vi "Begin.vi"(8 "error in":errorcluster) -> (0 "error out":errorcluster)   [LabVIEW 2020]
doc: "Called before other user functions, this VI is expected to open initial I/O refnums, load in file data, and do all program initialization. Notice that the <B>error out</B> terminal is simply used for data flow. Wiring it to other structures or subVIs ensures that this VI runs first."
uses:
  <vilib>/Rock Robotics/WPI/DriverStation/WPI_DriverStationRobotMode2.ctl
  <vilib>/Rock Robotics/WPI/Joystick/WPI_JoystickDeviceEnum.ctl
  <vilib>/Rock Robotics/WPI/Solenoid/WPI_SolenoidChannel.ctl
  <vilib>/Rock Robotics/WPI/ThirdParty/Phoenix-LabVIEW/Motor Controller/Controls/CTRE_Phoenix_MotorControl_NeutralMode.ctl
  <vilib>/Rock Robotics/SystemInterfaces/DIO/FPGA_DIOChannel.ctl
  Status Frame Stuff/Talon Status Config Array.ctl
  Status Frame Stuff/Talon Status Frame Setting.ctl
  <vilib>/Rock Robotics/WPI/ThirdParty/Phoenix-LabVIEW/Motor Controller/Controls/CTRE_Phoenix_MotorControl_StatusFrameEnhanced.ctl
  Status Frame Stuff/STATUS_Period.ctl
  Status Frame Stuff/Pigeon Status Config Array.ctl
  <vilib>/Rock Robotics/WPI/ThirdParty/Phoenix-LabVIEW/Pigeon IMU/CTRE_PigeonIMU_StatusFrameRate.ctl
  <vilib>/Rock Robotics/WPI/ThirdParty/REV Robotics/REVLib/Typedef/Spark MAX Idle Mode.ctl
  Robot Global Data.vi
  <vilib>/Rock Robotics/WPI/Utilities/WPI_GetSetVariantRefNum.vi
  <vilib>/Rock Robotics/WPI/Solenoid/WPI_SolenoidOpenDouble.vi
  <vilib>/Rock Robotics/WPI/ThirdParty/Phoenix-LabVIEW/Pigeon IMU/CTRE_PigeonIMU_Open_CAN.vi
panel:
  in  "Flywheel PIDF Constants":T1={"Set Constants"=TRUE, "P"=0.1, "I"=0.001, "D"=0.0, "F"=0.0461, "I Zone"=1000.0, "Cruise Velocity"=0, "Acceleration"=0, "Percent Deadband"=0.0}
  in  "Climber PIDF":T1={"Set Constants"=TRUE, "P"=0.45, "I"=0.0, "D"=0.0, "F"=0.0, "I Zone"=0.0, "Cruise Velocity"=20000, "Acceleration"=40000, "Percent Deadband"=0.7}
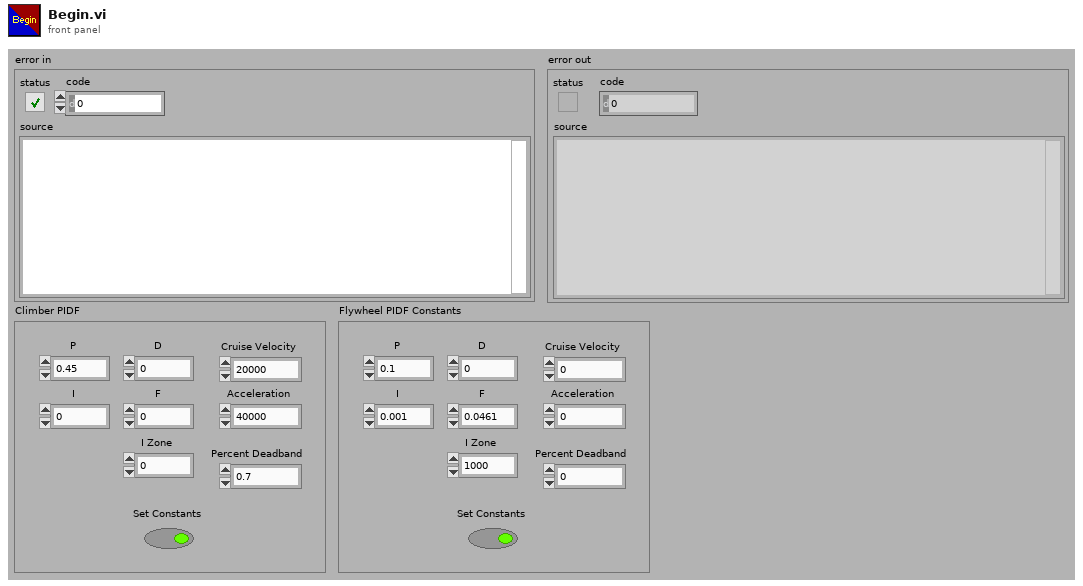
[diagram p1: front panel]
types:
  T1 = cluster{"Set Constants":bool, "P":dbl, "I":dbl, "D":dbl, "F":dbl, "I Zone":dbl, "Cruise Velocity":i32, "Acceleration":i32, "Percent Deadband":dbl}
  T2 = typedef "Pigeon Status Config Array.ctl" = cluster{"Status Frame Enum":T3, "STATUS_Period":T4}[]
  T3 = typedef "CTRE_PigeonIMU_StatusFrameRate.ctl" = u32
  T4 = typedef "STATUS_Period.ctl" = i32
  T5 = typedef "CTRE_Phoenix_MotorControl_NeutralMode.ctl" = enum8{"EEPROMSetting", "Override to Coast", "Override to Brake"}
  T6 = typedef "Talon Status Config Array.ctl" = T7[]
  T7 = typedef "Talon Status Frame Setting.ctl" = cluster{"Status Frame Enum":T8, "STATUS_Period":T4}
  T8 = typedef "CTRE_Phoenix_MotorControl_StatusFrameEnhanced.ctl" = u16
  T9 = typedef "FPGA_DIOChannel.ctl" = enum8{"DIO 0", "DIO 1", "DIO 2", "DIO 3", "DIO 4", "DIO 5", "DIO 6", "DIO 7", "DIO 8", "DIO 9", "DIO MXP 0", "DIO MXP 1", "DIO MXP 2", "DIO MXP 3", "DIO MXP 4", "DIO MXP 5", "DIO MXP 6", "DIO MXP 7", "DIO MXP 8", "DIO MXP 9", "DIO MXP 10", "DIO MXP 11", "DIO MXP 12", "DIO MXP 13", "DIO MXP 14", "DIO MXP 15", "SPI Port CS1", "SPI Port CS2", "SPI Port CS3", "SPI Port MISO", "SPI Port MOSI", "Invalid"}
  T10 = typedef "WPI_SolenoidChannel.ctl" = enum8{"Solenoid 0", "Solenoid 1", "Solenoid 2", "Solenoid 3", "Solenoid 4", "Solenoid 5", "Solenoid 6", "Solenoid 7", "Solenoid 8", "Solenoid 9", "Solenoid 10", "Solenoid 11", "Solenoid 12", "Solenoid 13", "Solenoid 14", "Solenoid 15", "Invalid"}
  T11 = typedef "WPI_JoystickDeviceEnum.ctl" = enum16{"USB 0", "USB 1", "USB 2", "USB 3", "USB 4", "USB 5"}
  T12 = typedef "WPI_DriverStationRobotMode2.ctl" = enum16{"Autonomous Disabled", "Autonomous Enabled", "Teleop Disabled", "Teleop Enabled", "Disconnected", "Finish", "Test Disabled", "Test Enabled", "Emergency Stopped"}
  T13 = typedef "WPI_JoystickDevRef.ctl" = cluster{"Device":T11}
  T14 = typedef "WPI_CompressorDevRef.ctl" = cluster{"DevStatus":errorcluster, "Pneumatics Control Module":u8}
  T15 = typedef "WPI_SolenoidDevRef.ctl" = cluster{"DevStatus":errorcluster, "Pneumatics Control Module":u8, "Forward Solenoid Channel":T10, "Reverse Solenoid Channel":T10}
  T16 = typedef "WPI_DigitalInputDevRef.ctl" = cluster{"DevStatus":errorcluster, "DIO Channel":T9}
  T17 = typedef "CTRE_PigeonIMU_DeviceRef.ctl" = cluster{"DeviceStatus":errorcluster, "Device Number":u8, "Type":T18, "Device ID":u32, "Handle":u64, "UsageFrame":u32, "Library Path":path}
  T18 = typedef "CTRE_PigeonIMU_ConnectionType.ctl" = u32
  T19 = typedef "WPI_MotorControlDeviceRef.ctl" = cluster{"DeviceStatus":errorcluster, "Type":T20, "PWM":cluster{"PWM Channel":T21, "DeadBand":T22}, "CAN":cluster{"Device Number":u8, "SetOutput VI Ref":variant, "GetOutput VI Ref":variant, "Enable VI Ref":variant, "Disable VI Ref":variant, "Data":variant}, "Invert":bool, "DIO PWM":cluster{"PWM \"Enable\" Channel":T21, "DIOChannel":T9, "PWM Rate":dbl}}
  T20 = typedef "WPI_MotorControlType.ctl" = enum16{"PWM", "CAN", "DIO PWM"}
  T21 = typedef "FPGA_DIOPWMChannel.ctl" = enum8{"PWM 0", "PWM 1", "PWM 2", "PWM 3", "PWM 4", "PWM 5", "PWM 6", "PWM 7", "PWM 8", "PWM 9", "PWM MXP 0", "PWM MXP 1", "PWM MXP 2", "PWM MXP 3", "PWM MXP 4", "PWM MXP 5", "PWM MXP 6", "PWM MXP 7", "PWM MXP 8", "PWM MXP 9", "Invalid"}
  T22 = typedef "WPI_PWMDeadband.ctl" = cluster{"Name":string, "maxPositivePwm":i32, "minPositivePwm":i32, "centerPwm":i32, "maxNegativePwm":i32, "minNegativePwm":i32, "angularRange":u16}
  T23 = typedef "Spark MAX Idle Mode.ctl" = enum16{"Coast", "Brake"}
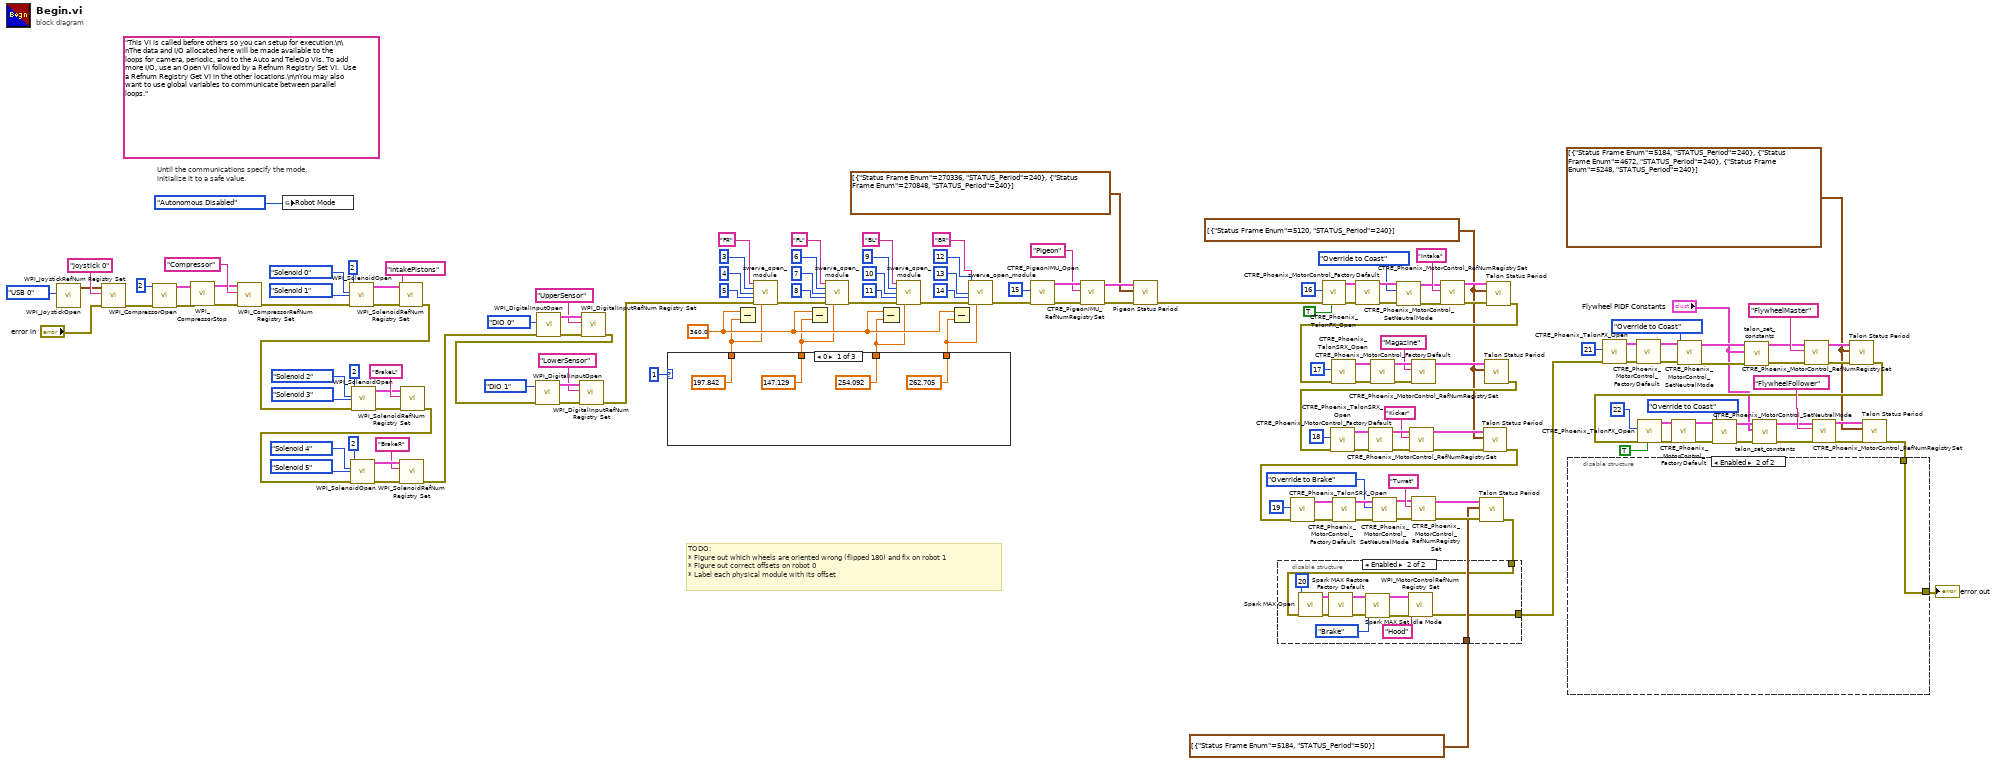
[diagram p0: block diagram]
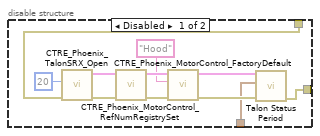
[diagram p2: hidden frame]
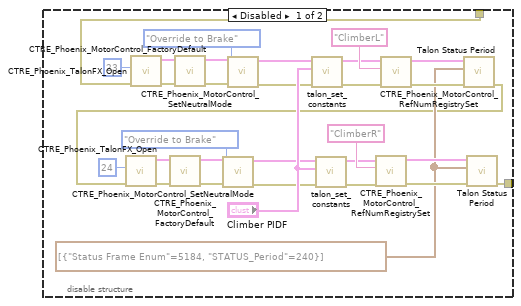
[diagram p3: hidden frame]
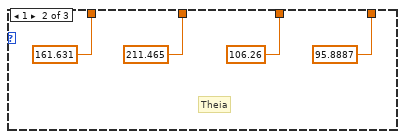
[diagram p4: hidden frame]
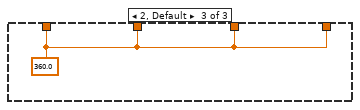
[diagram p5: hidden frame]
diagram:
  w30 = T6 [{"Status Frame Enum"=5184, "STATUS_Period"=240}, {"Status Frame Enum"=4672, "STATUS_Period"=240}, {"Status Frame Enum"=5248, "STATUS_Period"=240}] ("Drive Status Config")
  w31 = T6 [{"Status Frame Enum"=5184, "STATUS_Period"=50}] ("Drive Status Config")
  w32 = T6 [{"Status Frame Enum"=5120, "STATUS_Period"=240}] ("Drive Status Config")
  w127 = 360.0 ("Encoder Offset (Deg)")
  (unwired) "This VI is called before others so you can setup for execution.\n\nThe data and I/O allocated here will be made available to the loops for camera, periodic, and to the Auto and TeleOp VIs. To add more I/O, use an Open VI followed by a Refnum Registry Set VI.  Use a Refnum Registry Get VI in the other locations.\n\nYou may also want to use global variables to communicate between parallel loops."
  # "TODO:\n* Figure out which wheels are oriented wrong (flipped 180) and fix on robot 1\n* Figure out correct offsets on robot 0\n* Label each physical module with its offset"
  # "Until the communications specify the mode,\ninitialize it to a safe value."
  n1 = call <vilib>:"WPI_JoystickOpen.vi"("JoystickDevice"=WPI_JoystickDeviceEnum."USB 0") -> ("JoystickDevRef"=w153:T13)  [unwired: 10 in]
  n2 = call <vilib>:"WPI_JoystickRefNum Registry Set.vi"("error in (no error)"="error in", "refnum name"="Joystick 0", "JoystickDevRef"=w153) -> ("error out"=w71:errorcluster)  [unwired: 7 in, 1 out]
  n3 = call <vilib>:"WPI_CompressorOpen.vi"("Pneumatics device (def)"=u8 2, "error in (no error)"=w71) -> ("CompressorDevRef"=w24:T14, "error out"=w25:errorcluster)  [unwired: 12 in]
  n4 = call <vilib>:"WPI_CompressorStop.vi"("error in (no error)"=w25, "CompressorDevRef"=w24) -> ("error out"=w22:errorcluster, "CompressorDevRef"=w23:T14)  [unwired: 8 in]
  n5 = call <vilib>:"WPI_CompressorRefNum Registry Set.vi"("error in (no error)"=w22, "refnum name"="Compressor", "CompressorDevRef"=w23) -> ("error out"=w69:errorcluster)  [unwired: 7 in, 1 out]
  n6 = global write "Robot Global Data.vi" "Robot Mode"(WPI_DriverStationRobotMode2."Autonomous Disabled" ("Robot Mode")) -> ()
  n7 = call-poly <vilib>:"WPI_SolenoidOpen.vi"("error in (no error)"=w69, "Reverse Solenoid Channel"=WPI_SolenoidChannel."Solenoid 1", "Forward Solenoid Channel"=WPI_SolenoidChannel."Solenoid 0", "Pneumatics Device (def)"=u8 2) -> ("error out"=w126:errorcluster, "SolenoidDevRef"=w125:T15)  [unwired: 6 in]
  n8 = call <vilib>:"WPI_SolenoidRefNum Registry Set.vi"("error in (no error)"=w126, "refnum name"="IntakePistons", "SolenoidDevRef"=w125) -> ("error out"=w113:errorcluster)  [unwired: 7 in, 1 out]
  n9 = call-poly <vilib>:"WPI_SolenoidOpen.vi"("error in (no error)"=w113, "Reverse Solenoid Channel"=WPI_SolenoidChannel."Solenoid 3", "Forward Solenoid Channel"=WPI_SolenoidChannel."Solenoid 2", "Pneumatics Device (def)"=u8 2) -> ("error out"=w114:errorcluster, "SolenoidDevRef"=w115:T15)  [unwired: 6 in]
  n10 = call <vilib>:"WPI_SolenoidRefNum Registry Set.vi"("error in (no error)"=w114, "refnum name"="BrakeL", "SolenoidDevRef"=w115) -> ("error out"=w106:errorcluster)  [unwired: 7 in, 1 out]
  n11 = call-poly <vilib>:"WPI_SolenoidOpen.vi"("error in (no error)"=w106, "Reverse Solenoid Channel"=WPI_SolenoidChannel."Solenoid 5", "Forward Solenoid Channel"=WPI_SolenoidChannel."Solenoid 4", "Pneumatics Device (def)"=u8 2) -> ("error out"=w112:errorcluster, "SolenoidDevRef"=w111:T15)  [unwired: 6 in]
  n12 = call <vilib>:"WPI_SolenoidRefNum Registry Set.vi"("error in (no error)"=w112, "refnum name"="BrakeR", "SolenoidDevRef"=w111) -> ("error out"=w67:errorcluster)  [unwired: 7 in, 1 out]
  n13 = call <vilib>:"WPI_DigitalInputOpen.vi"("error in (no error)"=w67, "DIO Channel"=FPGA_DIOChannel."DIO 0") -> ("error out"=w80:errorcluster, "DigitalInputDevRef"=w79:T16)  [unwired: 8 in]
  n14 = call <vilib>:"WPI_DigitalInputRefNum Registry Set.vi"("error in (no error)"=w80, "refnum name"="UpperSensor", "DigitalInputDevRef"=w79) -> ("error out"=w75:errorcluster)  [unwired: 7 in, 1 out]
  n15 = call <vilib>:"WPI_DigitalInputOpen.vi"("error in (no error)"=w75, "DIO Channel"=FPGA_DIOChannel."DIO 1") -> ("error out"=w78:errorcluster, "DigitalInputDevRef"=w77:T16)  [unwired: 8 in]
  n16 = call <vilib>:"WPI_DigitalInputRefNum Registry Set.vi"("error in (no error)"=w78, "refnum name"="LowerSensor", "DigitalInputDevRef"=w77) -> ("error out"=w66:errorcluster)  [unwired: 7 in, 1 out]
  n17 = case shown="0" u8 1 ("Drive CAN ID") {
    tunnel: [197.842 ("Encoder Offset (Deg)") 161.631 ("Encoder Offset (Deg)") w164] -> w29
    tunnel: [147.129 ("Encoder Offset (Deg)") 211.465 ("Encoder Offset (Deg)") w164] -> w28
    tunnel: [254.092 ("Encoder Offset (Deg)") 106.26 ("Encoder Offset (Deg)") w164] -> w27
    tunnel: [262.705 ("Encoder Offset (Deg)") 95.8887 ("Encoder Offset (Deg)") w164] -> w26
    frame 0 {
    }
    frame 1 {
      # "Theia"
    }
    frame 2, Default {
      w164 = 360.0 ("Encoder Offset (Deg)")
    }
  }
  n18 = Subtract(x=w127, y=w29) -> ()  [unwired: 1 out]
  n19 = call "swerve_open_module.vi"("Module Suffix"="FR", "Drive CAN ID"=u8 3, "Azimuth CAN ID"=u8 4 ("Drive CAN ID"), "Encoder CAN ID"=u8 5 ("Drive CAN ID"), "error in"=w66, "Encoder Offset (Deg)"=w29) -> ("error out"=w140:errorcluster)  [unwired: 9 in]
  n20 = Subtract(x=w127, y=w28) -> ()  [unwired: 1 out]
  n21 = call "swerve_open_module.vi"("Module Suffix"="FL", "Drive CAN ID"=u8 6, "Azimuth CAN ID"=u8 7 ("Drive CAN ID"), "Encoder CAN ID"=u8 8 ("Drive CAN ID"), "error in"=w140, "Encoder Offset (Deg)"=w28) -> ("error out"=w135:errorcluster)  [unwired: 9 in]
  n22 = Subtract(x=w127, y=w27) -> ()  [unwired: 1 out]
  n23 = call "swerve_open_module.vi"("Module Suffix"="BL", "Drive CAN ID"=u8 9, "Azimuth CAN ID"=u8 10 ("Drive CAN ID"), "Encoder CAN ID"=u8 11 ("Drive CAN ID"), "error in"=w135, "Encoder Offset (Deg)"=w27) -> ("error out"=w130:errorcluster)  [unwired: 9 in]
  n24 = Subtract(x=w127, y=w26) -> ()  [unwired: 1 out]
  n25 = call "swerve_open_module.vi"("Module Suffix"="BR", "Drive CAN ID"=u8 12, "Azimuth CAN ID"=u8 13 ("Drive CAN ID"), "Encoder CAN ID"=u8 14 ("Drive CAN ID"), "error in"=w130, "Encoder Offset (Deg)"=w26) -> ("error out"=w128:errorcluster)  [unwired: 9 in]
  n26 = call-poly <vilib>:"CTRE_PigeonIMU_Open.vi"("error in"=w128, "Device Number"=u8 15) -> ("error out"=w150:errorcluster, "PigeonIMUDevRef"=w149:T17)  [unwired: 8 in]
  n27 = call <vilib>:"CTRE_PigeonIMU_RefNumRegistrySet.vi"("error in (no error)"=w150, "refnum name"="Pigeon", "PigeonIMUDevRef"=w149) -> ("error out"=w9:errorcluster, "PigeonIMUDevRef"=w10:T17)  [unwired: 7 in]
  n28 = call "Pigeon Status Period.vi"("error in (no error)"=w9, "Pigeon Status Config Array"=T2 [{"Status Frame Enum"=270336, "STATUS_Period"=240}, {"Status Frame Enum"=270848, "STATUS_Period"=240}], "PigeonIMUDevRef"=w10) -> ("error out"=w8:errorcluster)  [unwired: 7 in, 1 out]
  n29 = call <vilib>:"CTRE_Phoenix_TalonFX_Open.vi"("Invert"=TRUE, "error in"=w8, "Device Number"=u8 16) -> ("error out"=w105:errorcluster, "PhoenixMotorControlDevRef"=w104:T19)  [unwired: 7 in]
  n30 = call <vilib>:"CTRE_Phoenix_MotorControl_FactoryDefault.vi"("error in"=w105, "PhoenixMotorControlDevRef"=w104) -> ("error out"=w100:errorcluster, "PhoenixMotorControlDevRef"=w101:T19)  [unwired: 8 in]
  n31 = call <vilib>:"CTRE_Phoenix_MotorControl_SetNeutralMode.vi"("error in (no error)"=w100, "Motor Control Neutral Mode"=CTRE_Phoenix_MotorControl_NeutralMode."Override to Coast", "PhoenixMotorControlDevRef"=w101) -> ("error out"=w98:errorcluster, "PhoenixMotorControlDevRef"=w99:T19)  [unwired: 7 in]
  n32 = call <vilib>:"CTRE_Phoenix_MotorControl_RefNumRegistrySet.vi"("error in (no error)"=w98, "refnum name"="Intake", "PhoenixMotorControlDevRef"=w99) -> ("error out"=w64:errorcluster, "PhoenixMotorControlDevRef"=w65:T19)  [unwired: 7 in]
  n33 = call "Talon Status Period.vi"("error in (no error)"=w64, "Status Config Array"=w32, "PhoenixMotorControlDevRef"=w65) -> ("error out"=w63:errorcluster)  [unwired: 7 in, 1 out]
  n34 = call <vilib>:"CTRE_Phoenix_TalonSRX_Open.vi"("error in"=w63, "Device Number"=u8 17) -> ("error out"=w96:errorcluster, "PhoenixMotorControlDevRef"=w95:T19)  [unwired: 8 in]
  n35 = call <vilib>:"CTRE_Phoenix_MotorControl_FactoryDefault.vi"("error in"=w96, "PhoenixMotorControlDevRef"=w95) -> ("error out"=w90:errorcluster, "PhoenixMotorControlDevRef"=w89:T19)  [unwired: 8 in]
  n36 = call <vilib>:"CTRE_Phoenix_MotorControl_RefNumRegistrySet.vi"("error in (no error)"=w90, "refnum name"="Magazine", "PhoenixMotorControlDevRef"=w89) -> ("PhoenixMotorControlDevRef"=w62:T19)  [unwired: 7 in, 1 out]
  n37 = call "Talon Status Period.vi"("Status Config Array"=w32, "PhoenixMotorControlDevRef"=w62) -> ("error out"=w61:errorcluster)  [unwired: 8 in, 1 out]
  n38 = call <vilib>:"CTRE_Phoenix_TalonSRX_Open.vi"("error in"=w61, "Device Number"=u8 18) -> ("error out"=w94:errorcluster, "PhoenixMotorControlDevRef"=w93:T19)  [unwired: 8 in]
  n39 = call <vilib>:"CTRE_Phoenix_MotorControl_FactoryDefault.vi"("error in"=w94, "PhoenixMotorControlDevRef"=w93) -> ("error out"=w88:errorcluster, "PhoenixMotorControlDevRef"=w87:T19)  [unwired: 8 in]
  n40 = call <vilib>:"CTRE_Phoenix_MotorControl_RefNumRegistrySet.vi"("error in (no error)"=w88, "refnum name"="Kicker", "PhoenixMotorControlDevRef"=w87) -> ("error out"=w59:errorcluster, "PhoenixMotorControlDevRef"=w60:T19)  [unwired: 7 in]
  n41 = call "Talon Status Period.vi"("error in (no error)"=w59, "Status Config Array"=w32, "PhoenixMotorControlDevRef"=w60) -> ("error out"=w58:errorcluster)  [unwired: 7 in, 1 out]
  n42 = call <vilib>:"CTRE_Phoenix_TalonSRX_Open.vi"("error in"=w58, "Device Number"=u8 19) -> ("error out"=w92:errorcluster, "PhoenixMotorControlDevRef"=w91:T19)  [unwired: 8 in]
  n43 = call <vilib>:"CTRE_Phoenix_MotorControl_FactoryDefault.vi"("error in"=w92, "PhoenixMotorControlDevRef"=w91) -> ("error out"=w17:errorcluster, "PhoenixMotorControlDevRef"=w20:T19)  [unwired: 8 in]
  n44 = call <vilib>:"CTRE_Phoenix_MotorControl_SetNeutralMode.vi"("error in (no error)"=w17, "Motor Control Neutral Mode"=CTRE_Phoenix_MotorControl_NeutralMode."Override to Brake", "PhoenixMotorControlDevRef"=w20) -> ("error out"=w18:errorcluster, "PhoenixMotorControlDevRef"=w19:T19)  [unwired: 7 in]
  n45 = call <vilib>:"CTRE_Phoenix_MotorControl_RefNumRegistrySet.vi"("error in (no error)"=w18, "refnum name"="Turret", "PhoenixMotorControlDevRef"=w19) -> ("error out"=w56:errorcluster, "PhoenixMotorControlDevRef"=w57:T19)  [unwired: 7 in]
  n46 = call "Talon Status Period.vi"("error in (no error)"=w56, "Status Config Array"=w31, "PhoenixMotorControlDevRef"=w57) -> ("error out"=w55:errorcluster)  [unwired: 7 in, 1 out]
  n47 = disable-structure shown="Enabled" {
    disable-tunnel: w55 -> [w169 w177]
    disable-tunnel: [w166 w179] -> w54
    disable-tunnel: w31 -> [w165 _]
    frame Disabled {
      n48 = call <vilib>:"CTRE_Phoenix_TalonSRX_Open.vi"("error in"=w169, "Device Number"=u8 20) -> ("error out"=w175:errorcluster, "PhoenixMotorControlDevRef"=w174:T19)  [unwired: 8 in]
      n49 = call <vilib>:"CTRE_Phoenix_MotorControl_FactoryDefault.vi"("error in"=w175, "PhoenixMotorControlDevRef"=w174) -> ("error out"=w173:errorcluster, "PhoenixMotorControlDevRef"=w172:T19)  [unwired: 8 in]
      n50 = call <vilib>:"CTRE_Phoenix_MotorControl_RefNumRegistrySet.vi"("error in (no error)"=w173, "refnum name"="Hood", "PhoenixMotorControlDevRef"=w172) -> ("error out"=w167:errorcluster, "PhoenixMotorControlDevRef"=w168:T19)  [unwired: 7 in]
      n51 = call "Talon Status Period.vi"("error in (no error)"=w167, "Status Config Array"=w165, "PhoenixMotorControlDevRef"=w168) -> ("error out"=w166:errorcluster)  [unwired: 7 in, 1 out]
    }
    frame Enabled {
      n52 = call <vilib>:"Spark MAX Open.vi"("error in (no error)"=w177, "Device Number"=u8 20) -> ("error out"=w186:errorcluster, "MotorControlDeviceRef"=w185:T19)  [unwired: 8 in]
      n53 = call <vilib>:"Spark MAX Restore Factory Default.vi"("error in"=w186, "MotorControlDeviceRef"=w185) -> ("error out"=w184:errorcluster, "MotorControlDeviceRef"=w183:T19)  [unwired: 8 in]
      n54 = call <vilib>:"Spark MAX Set Idle Mode.vi"("error in (no error)"=w184, "Idle Mode"=Spark_MAX_Idle_Mode."Brake", "MotorControlDeviceRef in"=w183) -> ("error out"=w180:errorcluster, "MotorControlDeviceRef out"=w181:T19)  [unwired: 7 in]
      n55 = call <vilib>:"WPI_MotorControlRefNum Registry Set.vi"("error in (no error)"=w180, "refnum name"="Hood", "MotorControlDevRef"=w181) -> ("error out"=w179:errorcluster)  [unwired: 7 in, 1 out]
    }
  }
  n56 = call <vilib>:"CTRE_Phoenix_TalonFX_Open.vi"("error in"=w54, "Device Number"=u8 21) -> ("error out"=w52:errorcluster, "PhoenixMotorControlDevRef"=w51:T19)  [unwired: 8 in]
  n57 = call <vilib>:"CTRE_Phoenix_MotorControl_FactoryDefault.vi"("error in"=w52, "PhoenixMotorControlDevRef"=w51) -> ("error out"=w47:errorcluster, "PhoenixMotorControlDevRef"=w48:T19)  [unwired: 8 in]
  n58 = call <vilib>:"CTRE_Phoenix_MotorControl_SetNeutralMode.vi"("error in (no error)"=w47, "Motor Control Neutral Mode"=CTRE_Phoenix_MotorControl_NeutralMode."Override to Coast", "PhoenixMotorControlDevRef"=w48) -> ("error out"=w12:errorcluster, "PhoenixMotorControlDevRef"=w15:T19)  [unwired: 7 in]
  n59 = call "talon_set_constants.vi"("error in"=w12, "Constants"="Flywheel PIDF Constants", "PhoenixMotorControlDevRef"=w15) -> ("error out"=w13:errorcluster, "PhoenixMotorControlDevRef"=w14:T19)  [unwired: 7 in]
  n60 = call <vilib>:"CTRE_Phoenix_MotorControl_RefNumRegistrySet.vi"("error in (no error)"=w13, "refnum name"="FlywheelMaster", "PhoenixMotorControlDevRef"=w14) -> ("error out"=w35:errorcluster, "PhoenixMotorControlDevRef"=w33:T19)  [unwired: 7 in]
  n61 = call "Talon Status Period.vi"("error in (no error)"=w35, "Status Config Array"=w30, "PhoenixMotorControlDevRef"=w33) -> ("error out"=w34:errorcluster)  [unwired: 7 in, 1 out]
  n62 = call <vilib>:"CTRE_Phoenix_TalonFX_Open.vi"("Invert"=TRUE, "error in"=w34, "Device Number"=u8 22) -> ("error out"=w45:errorcluster, "PhoenixMotorControlDevRef"=w44:T19)  [unwired: 7 in]
  n63 = call <vilib>:"CTRE_Phoenix_MotorControl_FactoryDefault.vi"("error in"=w45, "PhoenixMotorControlDevRef"=w44) -> ("error out"=w40:errorcluster, "PhoenixMotorControlDevRef"=w41:T19)  [unwired: 8 in]
  n64 = call <vilib>:"CTRE_Phoenix_MotorControl_SetNeutralMode.vi"("error in (no error)"=w40, "Motor Control Neutral Mode"=CTRE_Phoenix_MotorControl_NeutralMode."Override to Coast", "PhoenixMotorControlDevRef"=w41) -> ("error out"=w6:errorcluster, "PhoenixMotorControlDevRef"=w7:T19)  [unwired: 7 in]
  n65 = call "talon_set_constants.vi"("error in"=w6, "Constants"="Flywheel PIDF Constants", "PhoenixMotorControlDevRef"=w7) -> ("error out"=w4:errorcluster, "PhoenixMotorControlDevRef"=w5:T19)  [unwired: 7 in]
  n66 = call <vilib>:"CTRE_Phoenix_MotorControl_RefNumRegistrySet.vi"("error in (no error)"=w4, "refnum name"="FlywheelFollower", "PhoenixMotorControlDevRef"=w5) -> ("error out"=w36:errorcluster, "PhoenixMotorControlDevRef"=w37:T19)  [unwired: 7 in]
  n67 = call "Talon Status Period.vi"("error in (no error)"=w36, "Status Config Array"=w30, "PhoenixMotorControlDevRef"=w37) -> ("error out"=w3:errorcluster)  [unwired: 7 in, 1 out]
  n68 = disable-structure shown="Enabled" {
    disable-tunnel: [w217 w218] -> w53
    disable-tunnel: w3 -> [w187 w218]
    frame Disabled {
      w198 = T6 [{"Status Frame Enum"=5184, "STATUS_Period"=240}] ("Drive Status Config")
      n69 = call <vilib>:"CTRE_Phoenix_TalonFX_Open.vi"("error in"=w187, "Device Number"=u8 23) -> ("error out"=w216:errorcluster, "PhoenixMotorControlDevRef"=w215:T19)  [unwired: 8 in]
      n70 = call <vilib>:"CTRE_Phoenix_MotorControl_FactoryDefault.vi"("error in"=w216, "PhoenixMotorControlDevRef"=w215) -> ("error out"=w211:errorcluster, "PhoenixMotorControlDevRef"=w212:T19)  [unwired: 8 in]
      n71 = call <vilib>:"CTRE_Phoenix_MotorControl_SetNeutralMode.vi"("error in (no error)"=w211, "Motor Control Neutral Mode"=CTRE_Phoenix_MotorControl_NeutralMode."Override to Brake", "PhoenixMotorControlDevRef"=w212) -> ("error out"=w195:errorcluster, "PhoenixMotorControlDevRef"=w194:T19)  [unwired: 7 in]
      n72 = call "talon_set_constants.vi"("error in"=w195, "Constants"="Climber PIDF", "PhoenixMotorControlDevRef"=w194) -> ("error out"=w193:errorcluster, "PhoenixMotorControlDevRef"=w192:T19)  [unwired: 7 in]
      n73 = call <vilib>:"CTRE_Phoenix_MotorControl_RefNumRegistrySet.vi"("error in (no error)"=w193, "refnum name"="ClimberL", "PhoenixMotorControlDevRef"=w192) -> ("error out"=w201:errorcluster, "PhoenixMotorControlDevRef"=w202:T19)  [unwired: 7 in]
      n74 = call "Talon Status Period.vi"("error in (no error)"=w201, "Status Config Array"=w198, "PhoenixMotorControlDevRef"=w202) -> ("error out"=w191:errorcluster)  [unwired: 7 in, 1 out]
      n75 = call <vilib>:"CTRE_Phoenix_TalonFX_Open.vi"("error in"=w191, "Device Number"=u8 24) -> ("error out"=w209:errorcluster, "PhoenixMotorControlDevRef"=w208:T19)  [unwired: 8 in]
      n76 = call <vilib>:"CTRE_Phoenix_MotorControl_FactoryDefault.vi"("error in"=w209, "PhoenixMotorControlDevRef"=w208) -> ("error out"=w204:errorcluster, "PhoenixMotorControlDevRef"=w205:T19)  [unwired: 8 in]
      n77 = call <vilib>:"CTRE_Phoenix_MotorControl_SetNeutralMode.vi"("error in (no error)"=w204, "Motor Control Neutral Mode"=CTRE_Phoenix_MotorControl_NeutralMode."Override to Brake", "PhoenixMotorControlDevRef"=w205) -> ("error out"=w196:errorcluster, "PhoenixMotorControlDevRef"=w190:T19)  [unwired: 7 in]
      n78 = call "talon_set_constants.vi"("error in"=w196, "Constants"="Climber PIDF", "PhoenixMotorControlDevRef"=w190) -> ("error out"=w188:errorcluster, "PhoenixMotorControlDevRef"=w189:T19)  [unwired: 7 in]
      n79 = call <vilib>:"CTRE_Phoenix_MotorControl_RefNumRegistrySet.vi"("error in (no error)"=w188, "refnum name"="ClimberR", "PhoenixMotorControlDevRef"=w189) -> ("error out"=w199:errorcluster, "PhoenixMotorControlDevRef"=w200:T19)  [unwired: 7 in]
      n80 = call "Talon Status Period.vi"("error in (no error)"=w199, "Status Config Array"=w198, "PhoenixMotorControlDevRef"=w200) -> ("error out"=w217:errorcluster)  [unwired: 7 in, 1 out]
    }
    frame Enabled {
    }
  }
  "error out" <- w53
